vi "pmu_Phascale First 4 Bytes.vi"(7 "user designation":u8 format="%08b", 8 "error in (no error)":errorcluster, 9 "phasor phase":T1(ring), 10 "phasor unit":u32(ring) items=["Voltage [V]"=0, "Current [A]"=16777216], 11 "data modification flag":u16=1 format="%016b") -> (0 "error out":errorcluster, 3 "PHSCALE first 4 bytes":u32 format="%032b")   [LabVIEW 2013, in "NI_EP_PMU.lvlib"]
uses:
  <vilib>/addons/Electrical Power/PMU/NI_EP_PMU.lvlib
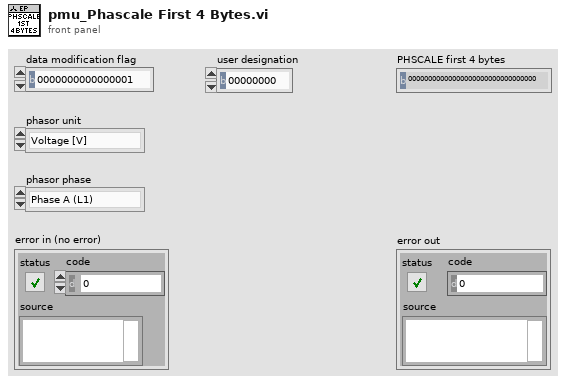
[diagram p1: front panel]
types:
  T1 = enum16{"Phase A (L1)", "Phase B (L2)", "Phase C (L3)", "Phase N", "Positive sequence", "Negative sequence", "Zero sequence"}
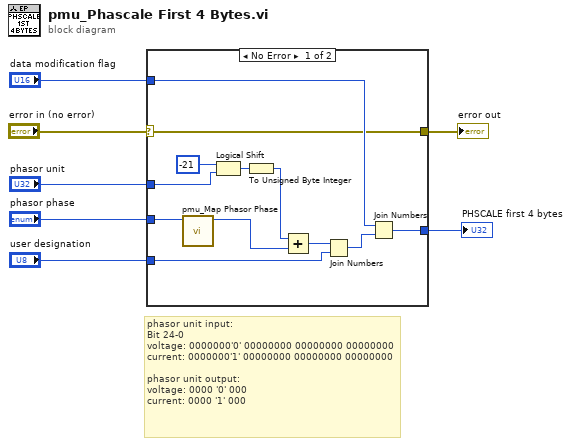
[diagram p0: block diagram]
diagram:
  # "phasor unit input:\nBit 24-0\nvoltage: 0000000'0' 00000000 00000000 00000000\ncurrent: 0000000'1' 00000000 00000000 00000000\n\nphasor unit output:\nvoltage: 0000 '0' 000\ncurrent: 0000 '1' 000"
  n1 = case shown="No Error" "error in (no error)" {
    selector: "error in (no error)" -> [w8 w20]
    tunnel: "data modification flag" -> [w9 _]
    tunnel: "phasor unit" -> [w12 _]
    tunnel: "phasor phase" -> [w14 _]
    tunnel: "user designation" -> [w18 _]
    tunnel: [w8 w20] -> w3
    tunnel: [w19 _] -> w2
    frame No Error {
      n2 = call <vilib>:"pmu_Map Phasor Phase.vi"("phasor phase in"=w14) -> ("phasor phase out"=w13:u8)  [unwired: 10 in]
      n3 = Logical Shift(y=i16 -21, x=w12) -> (x << y=w15:u32)
      n4 = To Unsigned Byte Integer(number=w15) -> (unsigned 8bit integer=w10:u8)
      n5 = Add(x=w10, y=w13) -> (x+y=w16:u8)
      n6 = Join Numbers(hi=w16, lo=w18) -> ((hi.lo)=w17:u16)
      n7 = Join Numbers(hi=w9, lo=w17) -> ((hi.lo)=w19:u32)
    }
    frame Error {
    }
  }
  "PHSCALE first 4 bytes" <- w2
  "error out" <- w3
